vi "ReadHead.vi"(11 "Data":string) -> (0 "Layers":i32, 1 "Units":dbl, 2 "Off":u32, 3 "Strings":string[](array[string]))   [LabVIEW 2012]
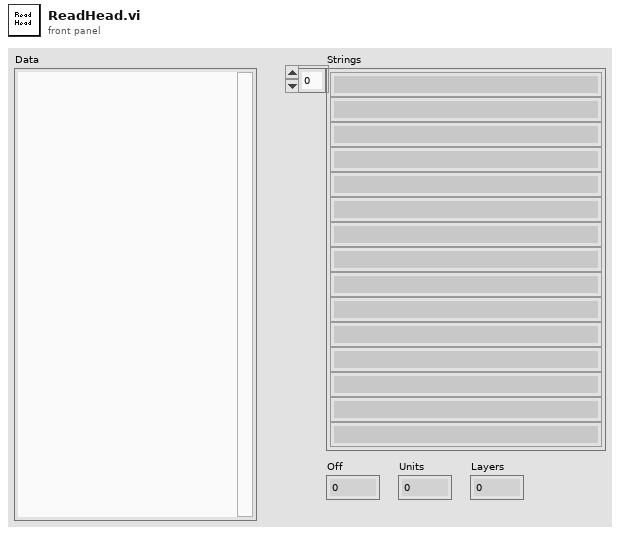
[diagram p1: front panel]
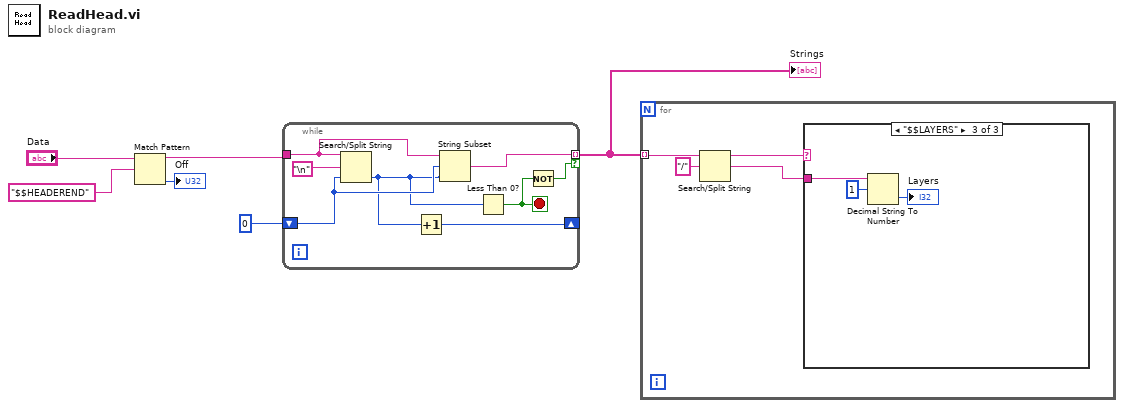
[diagram p0: block diagram]
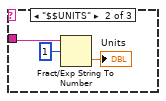
[diagram p3: hidden frame]
diagram:
  n1 = Match Pattern(string="Data", regular expression="$$HEADEREND" ("y")) -> (before substring=w3:string, offset past match=→"Off":i32)  [unwired: 1 in, 2 out]
  n2 = while {
    tunnel: w3 -> [w11]
    shift-right: [w13] -> _
    shift-left: 0 -> [w12]
    tunnel: [w10] -> w1 mode=indexing if=w7
    stop <- w8 stop-if-true
    n3 = Search/Split String(string=w11, search string/char (-)="\n", offset (0)=w12) -> (offset of match=w9:i32)  [unwired: 2 out]
    n4 = Increment(x=w9) -> (x+1=w13:i32)
    n5 = String Subset(string=w11, offset (0)=w12, length (rest)=w9) -> (substring=w10:string)
    n6 = Less Than 0?(x=w9) -> (x < 0?=w8:bool)
    n7 = Not(x=w8) -> (.not. x?=w7:bool)
  }
  "Strings" <- w1
  n8 = for {
    tunnel: w1 -> [w18] mode=indexing
    n9 = Search/Split String(string=w18, search string/char (-)="/") -> (substring before match=w16:string, match + rest of string=w15:string)  [unwired: 1 in, 1 out]
    n10 = case shown="\"$$LAYERS\"" w16 {
      tunnel: w15 -> [_ w21 w24]
      frame "\u0000", Default {
      }
      frame "$$UNITS" {
        n11 = Fract/Exp String To Number(string=w21, offset=1) -> (number=→"Units":dbl)  [unwired: 2 in, 1 out]
      }
      frame "$$LAYERS" {
        n12 = Decimal String To Number(string=w24, offset=1) -> (number=→"Layers":i32)  [unwired: 1 in, 1 out]
      }
    }
  }
